vi "ADXL.vi"() -> ()   [LabVIEW 2009]
panel:
  out "Total":dbl[](graph)
  out "Z":i32[](graph)
  out "Y":i32[](graph)
  out "X":i32[](graph)
  out "Z":i32[](array[numeric])
  out "Y":i32[](array[numeric])
  out "X":i32[](array[numeric])
  out "1/128 second":i32[](array[numeric])
  out "Second":i32[](array[numeric])
  out "Minute":i32[](array[numeric])
  out "Hour":i32[](array[numeric])
  out "Index":i32[](array[numeric])
  out "text":string
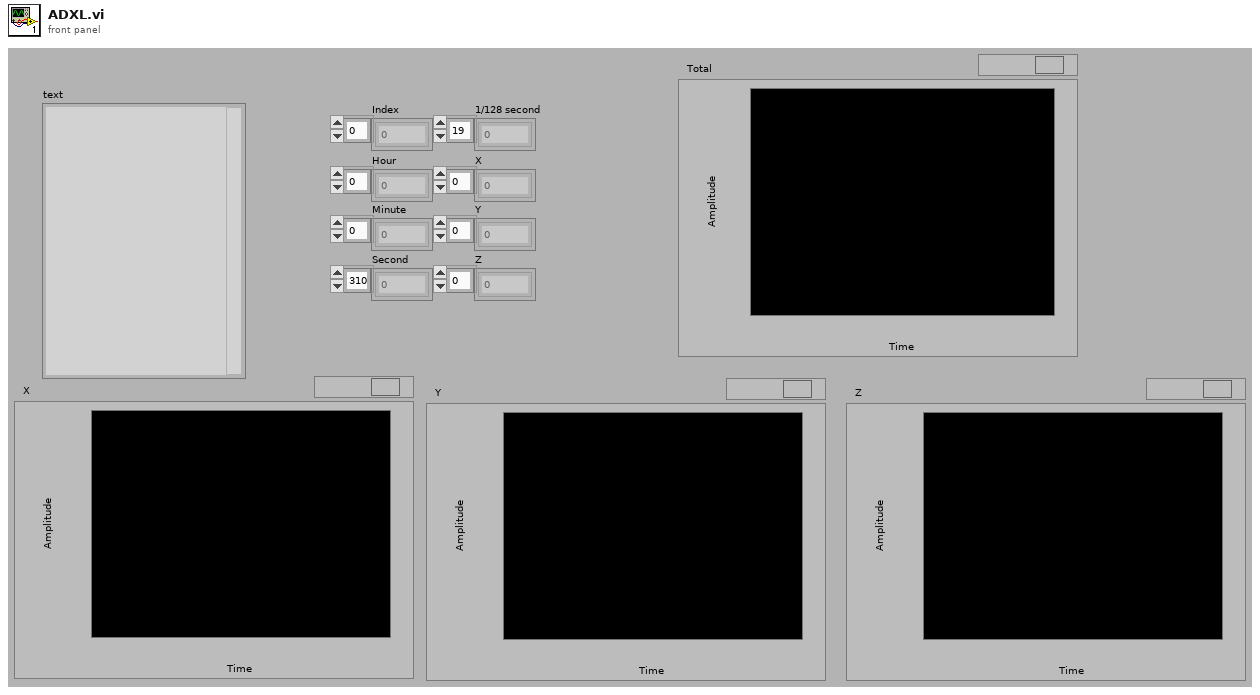
[diagram p1: front panel]
types:
  T1 = enum16{"open", "replace", "create", "open or create", "replace or create", "replace or create with confirmation"}
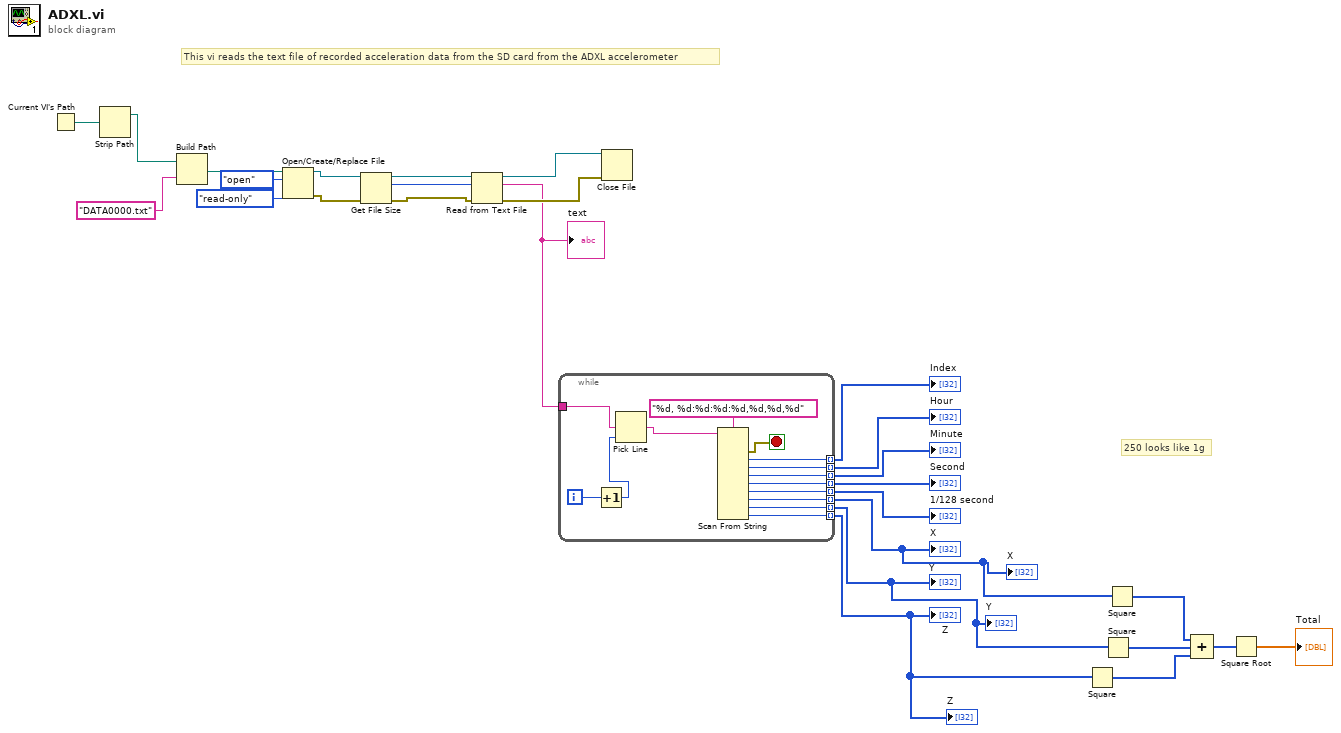
[diagram p0: block diagram]
diagram:
  # "This vi reads the text file of recorded acceleration data from the SD card from the ADXL accelerometer"
  # "250 looks like 1g"
  n1 = Current VI's Path() -> (path=w18:path)
  n2 = Strip Path(path=w18) -> (stripped path=w17:path)  [unwired: 1 out]
  n3 = Build Path(base path=w17, name or relative path="DATA0000.txt") -> (appended path=w26:path)
  n4 = Open/Create/Replace File(file path (use dialog)=w26, operation (0:open)=T1."open", access (0:read/write)=enum16{"read/write", "read-only", "write-only"}."read-only") -> (refnum out=w23:refnum<file>, error out=w22:errorcluster)  [unwired: 3 in, 1 out]
  n5 = Get File Size(file=w23, error in=w22) -> (refnum out=w21:refnum<file>, size (in bytes)=w14:i64, 0:w20:errorcluster)
  n6 = Read from Text File(file (use dialog)=w21, count=w14, error in=w20) -> (refnum out=w19:refnum<file>, text=w15:string, error out=w16:errorcluster)  [unwired: 1 in, 1 out]
  "text" <- w15
  n7 = while {
    tunnel: [w40] -> w13 mode=indexing
    tunnel: w15 -> [w37]
    tunnel: [w34] -> w12 mode=indexing
    tunnel: [w33] -> w11 mode=indexing
    tunnel: [w32] -> w10 mode=indexing
    tunnel: [w31] -> w9 mode=indexing
    tunnel: [w30] -> w8 mode=indexing
    tunnel: [w29] -> w7 mode=indexing
    tunnel: [w28] -> w6 mode=indexing
    i -> [w39]
    stop <- w35 stop-if-true
    n8 = Increment(x=w39) -> (x+1=w38:i32)
    n9 = Pick Line(multi-line string=w37, line index=w38) -> (output string=w36:string)  [unwired: 1 in]
    n10 = Scan From String(format string="%d, %d:%d:%d:%d,%d,%d,%d", input string=w36) -> (error out=w35:errorcluster, output 1=w40:i32, output 2=w34:i32, output 3=w33:i32, output 4=w32:i32, output 5=w31:i32, output 6=w30:i32, output 7=w29:i32, output 8=w28:i32)  [unwired: 10 in, 2 out]
  }
  "Index" <- w13
  "Hour" <- w12
  "Minute" <- w11
  "Second" <- w10
  "1/128 second" <- w9
  "X" <- w8
  "Y" <- w7
  "Z" <- w6
  "X" <- w8
  "Y" <- w7
  "Z" <- w6
  n11 = Close File(refnum=w19, error in=w16) -> ()  [unwired: 2 out]
  n12 = Square(x=w6) -> (x^2=w3:i32[])
  n13 = Square(x=w7) -> (x^2=w4:i32[])
  n14 = Square(x=w8) -> (x^2=w5:i32[])
  n15 = Compound Arithmetic op=ADD(w5, w4, w3) -> (w2:i32[])
  n16 = Square Root(x=w2) -> (sqrt(x)=→"Total":dbl[])
